vi "getStatus.vi"(0 "HGF_IMAQDevice":refnum<class "HGF_IMAQDevice.lvclass">, 5 "error in (no error)":errorcluster) -> (13 "Lost Counter":T1, 14 "dup HGF_IMAQDevice":refnum<class "HGF_IMAQDevice.lvclass">, 15 "Acquiring?":bool, 16 "Last Valid Buffer Index":u32, 17 "Last Valid Buffer Number":u32, 19 "error out":errorcluster)   [LabVIEW 2014, in "HGF_IMAQ.lvlib" / "HGF_IMAQDevice.lvclass"]
doc: "Returns status information about the acquisition, such as the state of the acquisition and the last valid buffer acquired."
uses:
  HGF_IMAQDevice.lvclass
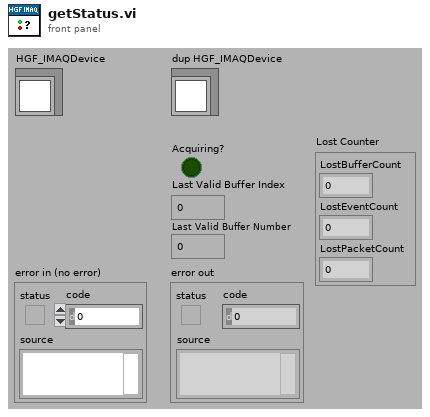
[diagram p1: front panel]
types:
  T1 = cluster{"LostBufferCount":u32, "LostEventCount":u32, "LostPacketCount":u32}
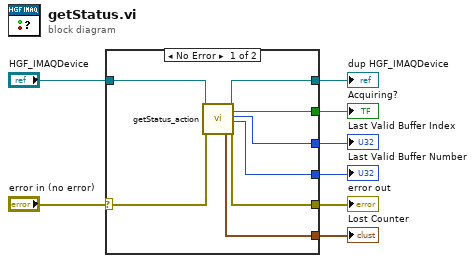
[diagram p0: block diagram]
diagram:
  n1 = case shown="No Error" "error in (no error)" {
    selector: "error in (no error)" -> [w14 w18]
    tunnel: [w13 w18] -> w7
    tunnel: [w15 w17] -> w5
    tunnel: "HGF_IMAQDevice" -> [w16 w17]
    tunnel: [w12 _] -> w4
    tunnel: [w11 _] -> w3
    tunnel: [w10 _] -> w2
    tunnel: [w9 _] -> w1
    frame No Error {
      n2 = call-dynamic "getStatus_action.vi"("HGF_IMAQDevice"=w16, "error in (no error)"=w14) -> ("Lost Counter"=w9:T1, "dup HGF_IMAQDevice"=w15:refnum<class "HGF_IMAQDevice.lvclass">, "Acquiring?"=w12:bool, "Last Valid Buffer Index"=w11:u32, "Last Valid Buffer Number"=w10:u32, "error out"=w13:errorcluster)  [unwired: 12 in]
    }
    frame Error {
    }
  }
  "error out" <- w7
  "dup HGF_IMAQDevice" <- w5
  "Acquiring?" <- w4
  "Last Valid Buffer Index" <- w3
  "Last Valid Buffer Number" <- w2
  "Lost Counter" <- w1
